vi "Setup.vi"(8 "error in (no error)":errorcluster, 11 "Process Test In":refnum<class "Person Test.lvclass">) -> (0 "error out":errorcluster, 3 "Process Test Out":refnum<class "Person Test.lvclass">)   [LabVIEW 2020, in "Person Test.lvclass"]
uses:
  Person Test.lvclass
  Processes/People/Person/Person.lvclass
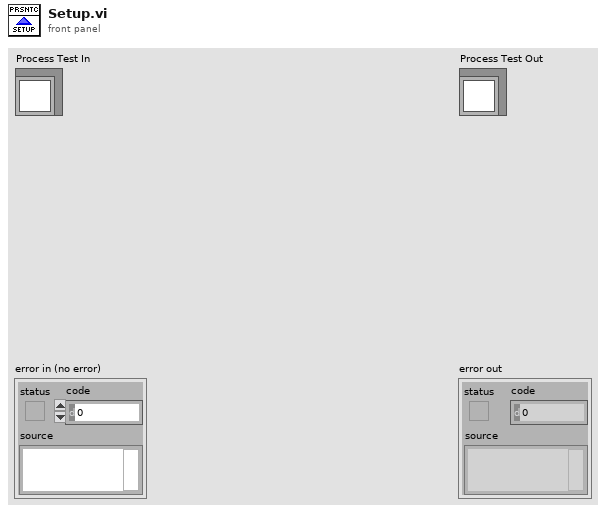
[diagram p1: front panel]
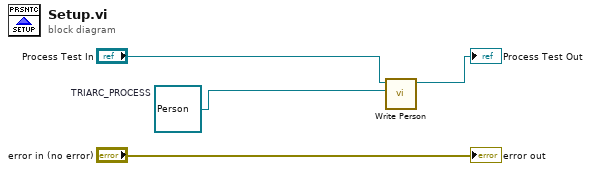
[diagram p0: block diagram]
diagram:
  w1 = refnum<class "Person.lvclass"> refnum  # TRIARC_PROCESS
  n1 = call "Write Person.vi"("TRIARC_PROCESS"=w1, "Person Test in"="Process Test In") -> ("Person Test out"=→"Process Test Out":refnum<class "Person Test.lvclass">)  [unwired: 9 in]
  "error out" <- "error in (no error)"
